vi "Trapezoidal Motion Profile.vi"(7 "Reset?":bool, 10 "Distance":dbl) -> (2 "Throttle Out":sgl, 4 "Finished?":bool)   [LabVIEW 2015]
uses:
  <vilib>/Rock Robotics/Network Tables/NT Read Number.vi
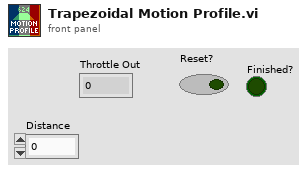
[diagram p1: front panel]
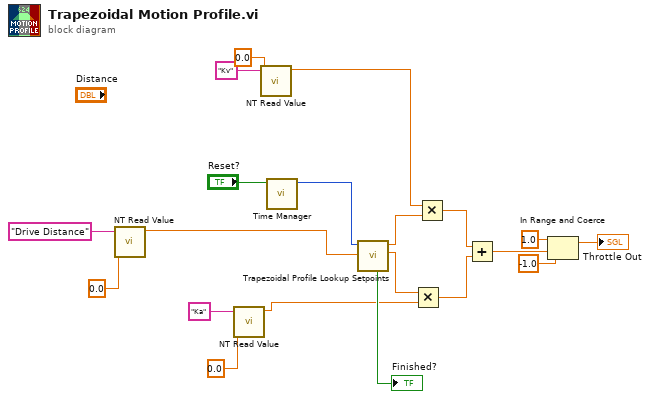
[diagram p0: block diagram]
diagram:
  n1 = call-poly <vilib>:"NT Read Value.vi"("Default Value"=0.0, "Name"="Drive Distance") -> ("Numeric"=w3:dbl)  [unwired: 8 in, 1 out]
  n2 = call-poly <vilib>:"NT Read Value.vi"("Default Value"=0.0, "Name"="Ka") -> ("Numeric"=w8:dbl)  [unwired: 8 in, 1 out]
  n3 = call-poly <vilib>:"NT Read Value.vi"("Default Value"=0.0, "Name"="Kv") -> ("Numeric"=w7:dbl)  [unwired: 8 in, 1 out]
  n4 = call "Time Manager.vi"("Reset?"="Reset?") -> ("Elapsed Time"=w19:u32)  [unwired: 10 in]
  n5 = call "Trapezoidal Profile Lookup Setpoints.vi"("Total Distance"=w3, "Current Time"=w19) -> ("Acceleration"=w12:sgl, "Velocity"=w11:sgl, "Profile Completed?"=→"Finished?":bool)  [unwired: 7 in]
  n6 = Multiply(x=w12, y=w8) -> (x*y=w13:dbl)
  n7 = Multiply(x=w7, y=w11) -> (x*y=w14:dbl)
  n8 = Add(x=w14, y=w13) -> (x+y=w15:dbl)
  n9 = In Range and Coerce(upper limit=sgl 1.0, x=w15, lower limit=sgl -1.0) -> (coerced(x)=→"Throttle Out":dbl)  [unwired: 1 out]
